vi "Actor Core.vi"(8 "error in":errorcluster, 11 "Python Protocol":refnum<class "Python Protocol.lvclass">) -> (0 "error out":errorcluster, 3 "Actor out":refnum<class "Actor.lvclass">)   [LabVIEW 2013, in "Python Protocol.lvlib" / "Python Protocol.lvclass"]
doc: "This is Actor Core.vi, the main message handling loop for Actors. An actor usually just sits in this loop and processes messages as they arrive. Any error returned by the message Do.vi call will stop the loop, with error code 43 as the canonical signal to stop with no error sent to caller. Descendants may override that in Handle Error.vi."
uses:
  Python Protocol.lvclass
  PluginInterface/Actor Framework.lvlibp/Actor/Actor.lvclass
  Python Protocol.lvclass/Python Protocol.ctl
  PluginInterface/PluginInterface.lvlibp/PluginInterfaceClass/PluginInterface.lvclass
  Python Protocol Messages/Change Status Msg/Change Status Msg.lvclass/Change Status Msg.ctl
  PluginInterface/Actor Framework.lvlibp/Message Enqueuer/Message Priority.ctl
  Write Start Time.vi
  Write Ring Refnum.vi
  Write Open.vi
  Write Save.vi
  Write Refresh.vi
  Write State.vi
  Write New.vi
  Write Path.vi
  Write Code.vi
  Write Compiler.vi
  PluginInterface/PluginInterface.lvlibp/PluginInterfaceClass/Write VI Refnum.vi
  PluginInterface/Actor Framework.lvlibp/Message Enqueuer/Enqueue.vi
  Python Protocol Messages/New Protocol Msg/New Protocol Msg.lvclass
  Python Protocol Messages/Open Protocol Msg/Open Protocol Msg.lvclass
  Python Protocol Messages/Save Protocol Msg/Save Protocol Msg.lvclass
  Python Protocol Messages/Compile Protocol Msg/Compile Protocol Msg.lvclass
  Python Protocol Messages/Change Status Msg/Change Status Msg.lvclass
  Python Protocol Messages/Insert Variable Msg/Insert Variable Msg.lvclass
  Python Protocol Messages/Show Variables/Show Variables Msg.lvclass
  Python Protocol Messages/Run Protocol Msg/Run Protocol Msg.lvclass
  PluginInterface/Actor Framework.lvlibp/Stop Msg/Stop Msg.lvclass
  PluginInterface/Actor Framework.lvlibp/Message Enqueuer/Message Enqueuer.lvclass
panel:
  in  "stop signal":bool
  in  "Menu Ring":u16(ring) items=["fgfdgdfgdfg", ""]
  in  "Radio Buttons":T1(radio)=enum."Media Stop Button"
  in  "Open Button":bool
  in  "New Button":bool
  in  "Refresh Button":bool
  in  "Save Button":bool
  out "File Path Control":path
  in  "Code":string
  out "Compiler":string
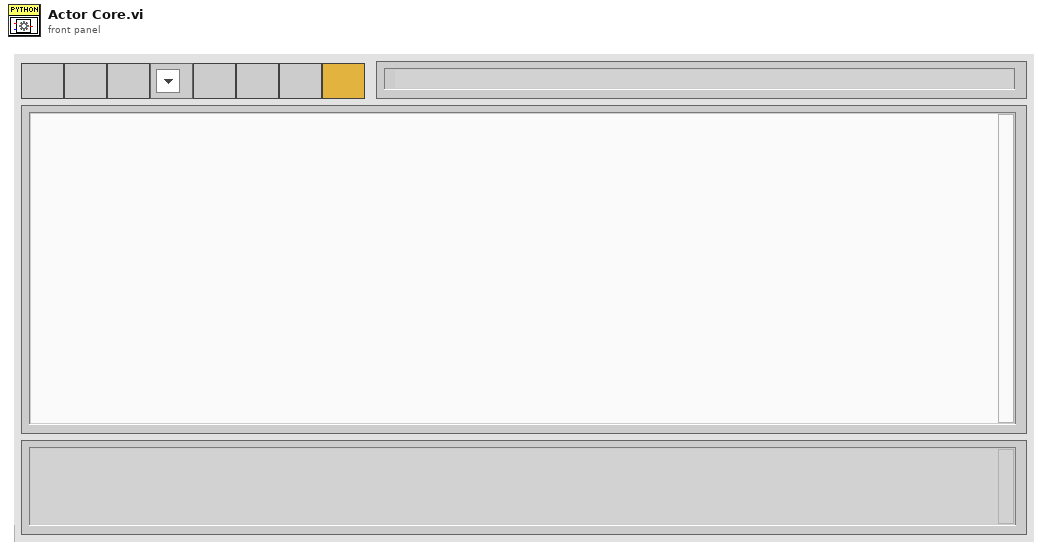
[diagram p1: front panel]
types:
  T1 = enum32{"Pause Button", "Play Button", "Media Stop Button"}
  T2 = typedef "Actor Framework.lvlibp/Message Enqueuer.lvclass/Message Priority.ctl" = enum16{"Low", "Normal", "High"}
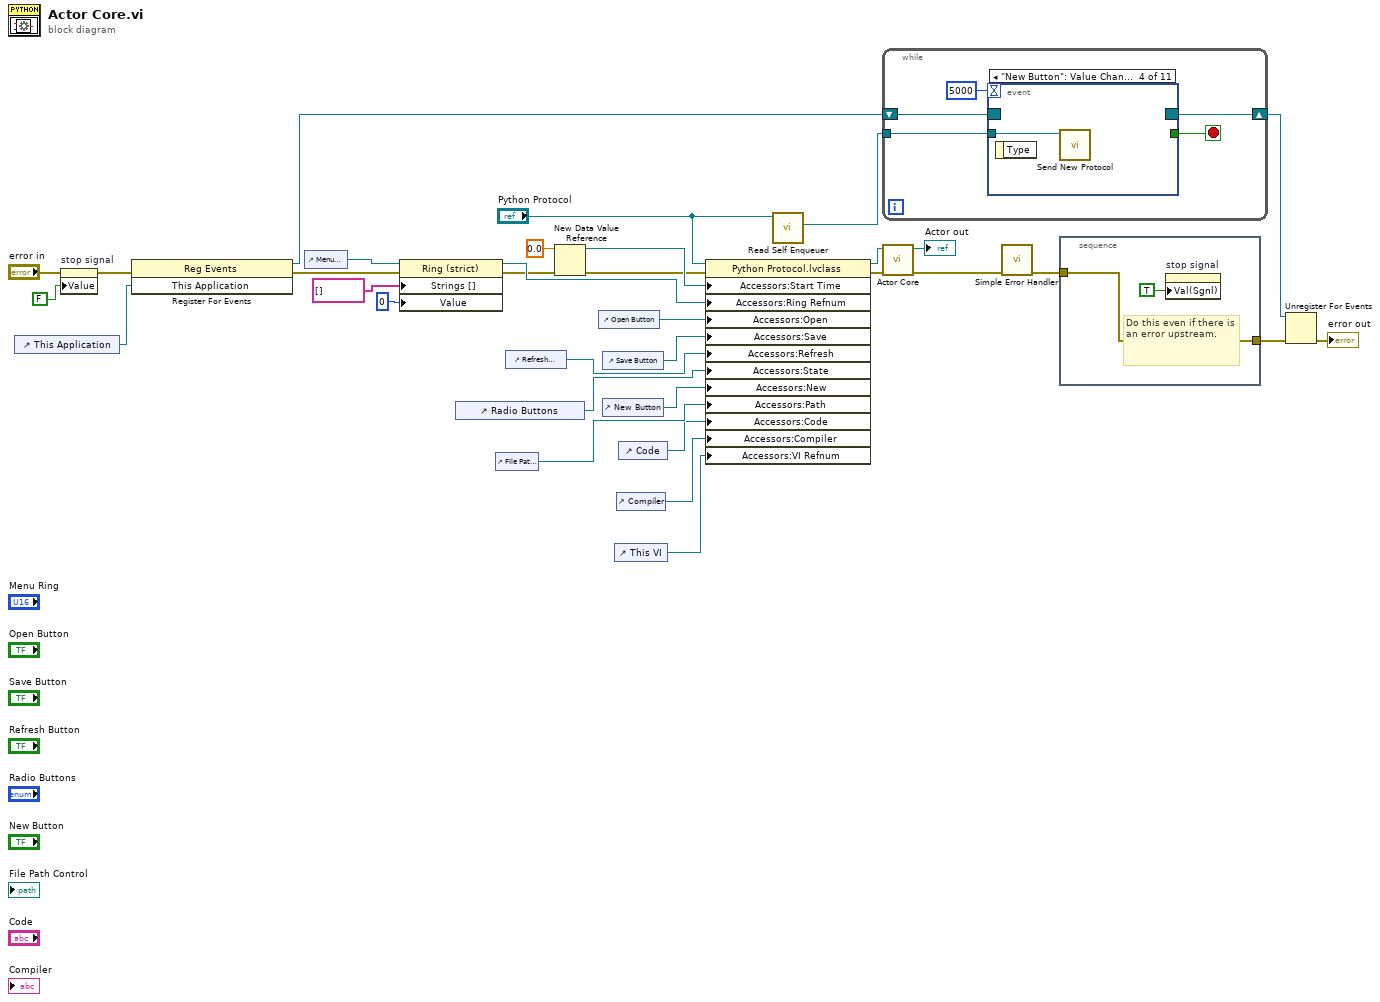
[diagram p0: block diagram]
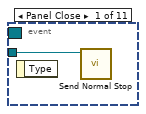
[diagram p2: hidden frame]
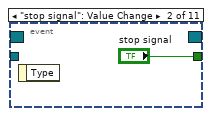
[diagram p3: hidden frame]
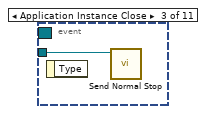
[diagram p4: hidden frame]
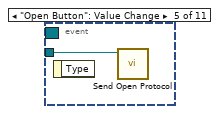
[diagram p5: hidden frame]
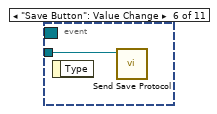
[diagram p6: hidden frame]
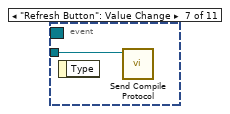
[diagram p7: hidden frame]
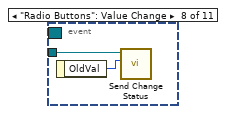
[diagram p8: hidden frame]
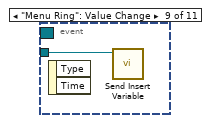
[diagram p9: hidden frame]
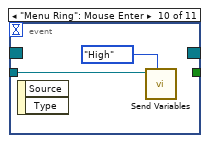
[diagram p10: hidden frame]
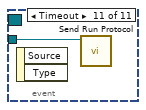
[diagram p11: hidden frame]
diagram:
  n1 = control-ref of="This Application"() -> (w26:refnum<vi>)
  n2 = property on="stop signal" class="Bool (strict)"(error in="error in", "Value"=FALSE ("stop")) -> (error out=w27:errorcluster)  [unwired: 1 in, 1 out]
  n3 = register-events(error in=w27, w26) -> (reference out=w30:refnum<event-registration>, error out=w5:errorcluster)  [unwired: 1 in]
  n4 = control-ref of="Menu Ring"() -> (w11:refnum<vi>)
  n5 = property class="Ring (strict)"(reference=w11, error in=w5, "Strings []"=string[] [], "Value"=u16 0) -> (reference out=w8:refnum<vi>, error out=w7:errorcluster)
  n6 = control-ref of="Radio Buttons"() -> (w19:refnum<vi>)
  n7 = control-ref of="File Path Control"() -> (w17:refnum<vi>)
  n8 = control-ref of="Refresh Button"() -> (w20:refnum<vi>)
  n9 = New Data Value Reference(data value=0.0, error in=w7) -> (data value reference=w4:refnum<data-value>, error out=w1:errorcluster)
  n10 = control-ref of="Open Button"() -> (w12:refnum<vi>)
  n11 = control-ref of="Save Button"() -> (w21:refnum<vi>)
  n12 = control-ref of="New Button"() -> (w18:refnum<vi>)
  n13 = control-ref of="This VI"() -> (w14:refnum<vi>)
  n14 = control-ref of="Compiler"() -> (w15:refnum<vi>)
  n15 = control-ref of="Code"() -> (w16:refnum<vi>)
  n16 = property class="Python Protocol.lvclass"(reference="Python Protocol", error in=w1, "Accessors:Start Time"=w4, "Accessors:Ring Refnum"=w8, "Accessors:Open"=w12, "Accessors:Save"=w21, "Accessors:Refresh"=w20, "Accessors:State"=w19, "Accessors:New"=w18, "Accessors:Path"=w17, "Accessors:Code"=w16, "Accessors:Compiler"=w15, "Accessors:VI Refnum"=w14) -> (reference out=w13:refnum<class "Python Protocol.lvclass">, error out=w25:errorcluster)
  n17 = call "Read Self Enqueuer.vi"("Actor"="Python Protocol") -> ("Self Enqueuer"=w2:refnum<class "Message Enqueuer.lvclass">)  [unwired: 10 in]
  n18 = while {
    tunnel: w2 -> [w38]
    shift-right: [w35] -> w29
    shift-left: w30 -> [w36]
    stop <- w37 stop-if-true
    n19 = event shown="[3] \"New Button\": Value Change" {
      selector: w36 -> [_ _ _ _ _ _ _ _ _ _ _]
      dyn-events: [_ _ _ _ _ _ _ _ _ _ _] -> w35
      timeout: 5000 -> [_ _ _ _ _ _ _ _ _ _ _]
      tunnel: w38 -> [w39 _ w41 w42 w43 w44 w45 w47 w48 w50 w51]
      tunnel: [_ "stop signal" _ _ _ _ _ _ _ _ _] -> w37
      event Panel Close {
        n20 = event-data() -> ()  [unwired: 1 in, 1 out]
        n21 = call "Send Normal Stop.vi"("Message Enqueuer"=w39) -> ()  [unwired: 10 in, 1 out]
      }
      event "stop signal": Value Change {
        n22 = event-data() -> ()  [unwired: 1 in, 1 out]
      }
      event Application Instance Close {
        n23 = event-data() -> ()  [unwired: 1 in, 1 out]
        n24 = call "Send Normal Stop.vi"("Message Enqueuer"=w41) -> ()  [unwired: 10 in, 1 out]
      }
      event "New Button": Value Change {
        n25 = event-data() -> ()  [unwired: 1 in, 1 out]
        n26 = call "Send New Protocol.vi"("Message Enqueuer"=w42) -> ()  [unwired: 9 in, 2 out]
      }
      event "Open Button": Value Change {
        n27 = event-data() -> ()  [unwired: 1 in, 1 out]
        n28 = call "Send Open Protocol.vi"("Message Enqueuer"=w43) -> ()  [unwired: 9 in, 2 out]
      }
      event "Save Button": Value Change {
        n29 = event-data() -> ()  [unwired: 1 in, 1 out]
        n30 = call "Send Save Protocol.vi"("Message Enqueuer"=w44) -> ()  [unwired: 9 in, 2 out]
      }
      event "Refresh Button": Value Change {
        n31 = event-data() -> ()  [unwired: 1 in, 1 out]
        n32 = call "Send Compile Protocol.vi"("Message Enqueuer"=w45) -> ()  [unwired: 9 in, 2 out]
      }
      event "Radio Buttons": Value Change {
        n33 = event-data() -> ("OldVal"=w46:T1)  [unwired: 1 in]
        n34 = call "Send Change Status.vi"("Old Value"=w46, "Message Enqueuer"=w47) -> ()  [unwired: 8 in, 2 out]
      }
      event "Menu Ring": Value Change {
        n35 = event-data() -> ()  [unwired: 1 in, 2 out]
        n36 = call "Send Insert Variable.vi"("Message Enqueuer"=w48) -> ()  [unwired: 9 in, 2 out]
      }
      event "Menu Ring": Mouse Enter {
        n37 = event-data() -> ()  [unwired: 1 in, 2 out]
        n38 = call "Send Variables.vi"("Message Priority (Normal)"=Message_Priority."High", "Message Enqueuer"=w50) -> ()  [unwired: 8 in, 2 out]
      }
      event Timeout {
        n39 = event-data() -> ()  [unwired: 1 in, 2 out]
        n40 = call "Send Run Protocol.vi"("Message Enqueuer"=w51) -> ()  [unwired: 9 in, 2 out]
      }
    }
  }
  n41 = call-parent "Actor Core.vi"("error in"=w25, "Actor in"=w13) -> ("error out"=w32:errorcluster, "Actor out"=→"Actor out":refnum<class "Actor.lvclass">)  [unwired: 8 in]
  n42 = call <vilib>:"Simple Error Handler.vi"("error in (no error)"=w32) -> ("error out"=w31:errorcluster)  [unwired: 4 in, 4 out]
  n43 = stacked-sequence {
    tunnel: [w52] -> w28
    tunnel: w31 -> [w52]
    frame #0 {
      # "Do this even if there is an error upstream."
      n44 = property on="stop signal" class="Bool (strict)"("Val(Sgnl)"=TRUE ("stop")) -> ()  [unwired: 2 in, 2 out]
    }
  }
  n45 = Unregister For Events(event registration refnum=w29, error in=w28) -> (error out=→"error out":errorcluster)
